vi "Error.vi"(8 "Output 信息ERROR":string[](array[string]), 9 "Input 信息ERROR":string[](array[string]), 10 "轴信息ERROR":string[](array[string])) -> (2 "ERROR":string[](array[string]))   [LabVIEW 2012]
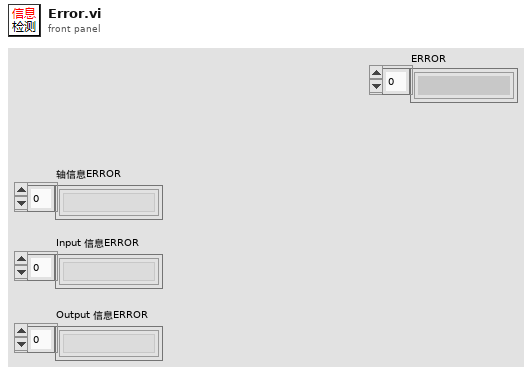
[diagram p1: front panel]
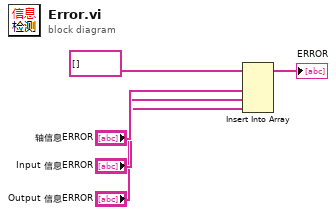
[diagram p0: block diagram]
diagram:
  n1 = Insert Into Array(array=string[] [], new element #1="轴信息ERROR", new element #2="Input 信息ERROR", new element #3="Output 信息ERROR") -> (→"ERROR":string[])  [unwired: 1 in]
